vi "_Add Argument.vi"(7 "Overwrite? (F)":bool, 8 "error in (no error)":errorcluster, 9 "Value":variant, 10 "Name":string, 11 "Arguments in":refnum<class "Values.lvclass">) -> (0 "error out":errorcluster, 3 "Arguments out":refnum<class "Values.lvclass">)   [LabVIEW 2020, in "HTTP Server.lvlib" / "Values.lvclass"]
uses:
  Values.lvclass
  Values.lvclass/Values.ctl
  <vilib>/Utility/miscctls.llb/LVMapReplaceAction.ctl
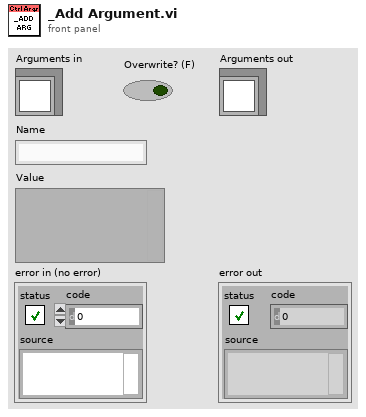
[diagram p1: front panel]
types:
  T1 = typedef "LVMapReplaceAction.ctl" = enum32{"Modify Entry only if found", "Add or Modify Entry", "Delete Entry"}
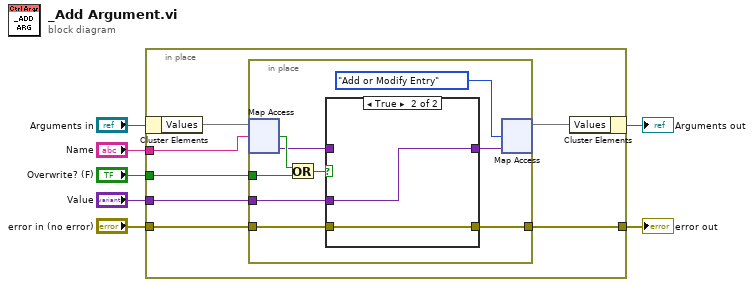
[diagram p0: block diagram]
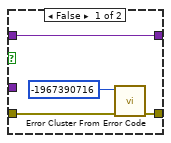
[diagram p2: hidden frame]
diagram:
  n1 = in-place {
    in-place-border: "Name" -> [w13]
    in-place-border: "Value" -> [w11]
    in-place-border: "Overwrite? (F)" -> [w12]
    in-place-border: "error in (no error)" -> [w10]
    in-place-border: [w9] -> w1
    n2 = in-place-cluster #1("Arguments in") -> ("Values"=w14:map{string, variant})
    n3 = in-place {
      in-place-border: w12 -> [w23]
      in-place-border: w11 -> [w17]
      in-place-border: w10 -> [w16]
      in-place-border: [w15] -> w9
      n4 = in-place-map #2(w14, w13) -> (w20:variant, w22:bool)  [unwired: 1 in]
      n5 = Or(x=w22, y=w23) -> (x .or. y?=w21:bool)
      n6 = case shown="True" w21 {
        tunnel: w20 -> [w27 _]
        tunnel: [w27 w29] -> w19
        tunnel: w17 -> [_ w29]
        tunnel: w16 -> [w26 w28]
        tunnel: [w25 w28] -> w15
        frame False {
          n7 = call <vilib>:"Error Cluster From Error Code.vi"("error in (no error)"=w26, "error code (0)"=-1967390716) -> ("error out"=w25:errorcluster)  [unwired: 7 in]
        }
        frame True {
        }
      }
      n8 = in-place-map #2(w19, LVMapReplaceAction."Add or Modify Entry" ("action")) -> (w8:map{string, variant})  [unwired: 2 out]
    }
    n9 = in-place-cluster #1("Values"=w8) -> (→"Arguments out":refnum<class "Values.lvclass">)
  }
  "error out" <- w1
